vi "test Abort All.vi"(11 "Test Case In":refnum<class "Tests Event MessengerM.lvclass">) -> (0 "error out":errorcluster, 3 "Test Case Out":refnum<class "Tests Event MessengerM.lvclass">)   [LabVIEW 2020, in "Tests Event MessengerM.lvclass"]
uses:
  Tests Event MessengerM.lvclass
  C:/Program Files/National Instruments/LabVIEW 2020/vi.lib/Astemes/LUnit/Test Case.lvclass
  <vilib>/Astemes/LUnit/Test Case.lvclass/Test Case.ctl
  <vilib>/Astemes/LUnit/Core/LUnit Test Case/Private/Append Fail Result.vi
  <vilib>/Astemes/LUnit/Core/LUnit Test Case/Private/Append Pass Result.vi
  <vilib>/Astemes/LUnit/Core/LUnit Test Case/Private/Run In UI.vi
  <vilib>/Utility/error.llb/Clear Errors.vi
  <extravilib>/ChannelInstances/Event MessengerM-c(str,var)/Instantiate.vi
  <extravilib>/ChannelInstances/Event MessengerM-c(str,var)/))Channel.vi
  Tests Event MessengerM.lvclass/Tests Event MessengerM.ctl
  <vilib>/Astemes/LUnit/Test Case.lvclass
  <extravilib>/ChannelInstances/Event MessengerM-c(str,var).lvlib
panel:
  out "cmd 2":string
  out "cmd":string
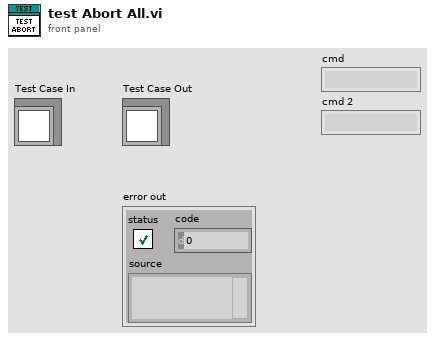
[diagram p1: front panel]
types:
  T1 = typedef "Event MessengerM-c(str,var).lvlib/))Channel.ctl" = refnum<queue>
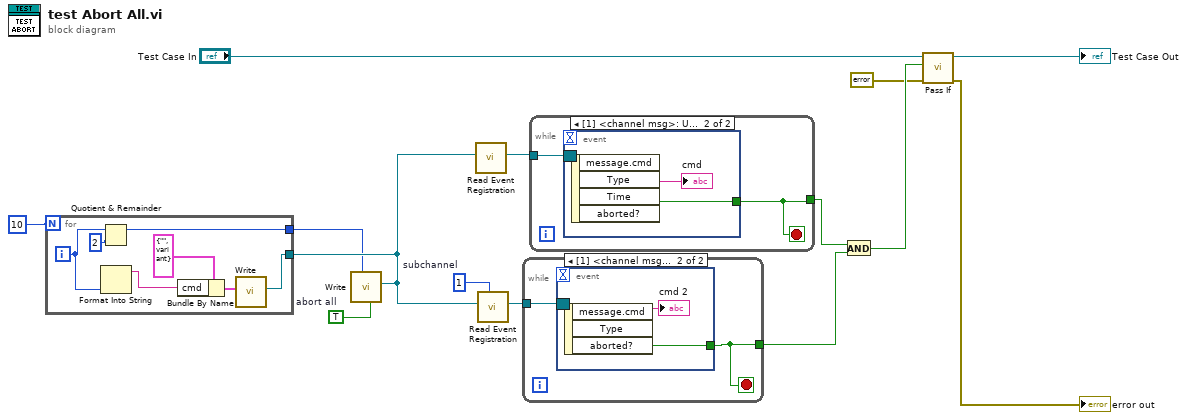
[diagram p0: block diagram]
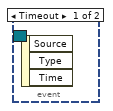
[diagram p2: hidden frame]
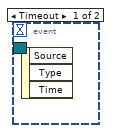
[diagram p3: hidden frame]
diagram:
  w5 = TRUE  # abort all
  w2 = 1  # subchannel
  n1 = for {
    N: 10 -> [_]
    tunnel: [w15] -> w6
    tunnel: [w17] -> w4
    i -> [w19]
    n2 = Quotient & Remainder(x=w19, y=2) -> (x-y*floor(x/y)=w17:i32)  [unwired: 1 out]
    n3 = Format Into String(w19) -> (resulting string=w18:string)  [unwired: 3 in, 1 out]
    n4 = Bundle By Name(cluster=cluster{"cmd":string, "data":variant} {"cmd"="", "data"=variant} ("element"), "cmd"=w18) -> (w16:cluster{"cmd":string, "data":variant})
    n5 = call <extravilib>:"Write.vi"("element"=w16) -> ("channel"=w15:T1)  [unwired: 9 in, 1 out]
  }
  n6 = call <extravilib>:"Write.vi"("channel"=w6, "abort all (F)"=w5, "subchannel (0)"=w4) -> ()  [unwired: 8 in, 1 out]
  n7 = call <extravilib>:"Read Event Registration.vi"("channel"=w6) -> ("event registration refnum"=w7:refnum<event-registration>)  [unwired: 10 in]
  n8 = call <extravilib>:"Read Event Registration.vi"("subchannel (0)"=w2, "channel"=w6) -> ("event registration refnum"=w3:refnum<event-registration>)  [unwired: 9 in]
  n9 = while {
    tunnel: w3 -> [w23]
    tunnel: [w22] -> w9
    stop <- w22 stop-if-true
    n10 = event shown="[1] <channel msg>: User Event" {
      selector: w23 -> [_ _]
      dyn-events: _ -> [_ _]
      timeout: _ -> [_ _]
      tunnel: [_ w24] -> w22
      event Timeout {
        n11 = event-data() -> ()  [unwired: 1 in, 3 out]
      }
      event User Event {
        n12 = event-data() -> ("message.cmd"=→"cmd 2":string, "aborted?"=w24:bool)  [unwired: 1 in, 1 out]
      }
    }
  }
  n13 = while {
    tunnel: w7 -> [w27]
    tunnel: [w26] -> w8
    stop <- w26 stop-if-true
    n14 = event shown="[1] <channel msg>: User Event" {
      selector: w27 -> [_ _]
      dyn-events: _ -> [_ _]
      timeout: _ -> [_ _]
      tunnel: [_ w29] -> w26
      event Timeout {
        n15 = event-data() -> ()  [unwired: 1 in, 3 out]
      }
      event User Event {
        n16 = event-data() -> ("message.cmd"=→"cmd":string, "aborted?"=w29:bool)  [unwired: 1 in, 2 out]
      }
    }
  }
  n17 = And(x=w8, y=w9) -> (x .and. y?=w10:bool)
  n18 = call <vilib>:"Pass If.vi"("error in (no error)"=errorcluster {"status"=FALSE, "code"=0, "source"=""}, "Pass?"=w10, "LUnit Test Case In"="Test Case In") -> ("error out"=→"error out":errorcluster, "LUnit Test Case Out"=→"Test Case Out":refnum<class "Tests Event MessengerM.lvclass">)  [unwired: 7 in]
